vi "Soft_Robot Model Two States.vi"() -> ()   [LabVIEW 2015]
uses:
  <vilib>/addons/Control Design/_Model Construction/Model Typedefs.llb/CD State Space Model (MIMO).ctl
  <vilib>/addons/Control Design/_Model Construction/Model Typedefs.llb/CD General Elements.ctl
  <vilib>/Analysis/7linalg.llb/Create Special Real Matrix.vi
  <vilib>/addons/Control Design/_Model Construction/Model Creation.llb/Model Creation SubVI/cd_Create State Space Model.vi
  <vilib>/addons/Control Design/_State Feedback Control/State Feedback Control.llb/State Feedback Control SubVis/cd_Linear Quadratic Regulator.vi
  <vilib>/addons/Control Design/_Stochastic Systems/Stochastic Systems.llb/CD Construct Noise Model (Numeric).vi
  <vilib>/Simulation/Estimation/Implementation/NILVSim Discrete Kalman Filter.llb/SIM Disc KF Pred and Corr with Pred Gain with Checking Direct LV.vi
  <vilib>/FPGAPlugInAG/myRIO-1900/niLvFpga_Open_myRIO-1900.vi
  <vilib>/rvi/interface/common/dynamic/niFpgaDynamicAddResources.vi
  <vilib>/Utility/error.llb/Error Cluster From Error Code.vi
  <vilib>/rvi/errors/niLvFpgaAdjustHostInterfaceError.vi
  <vilib>/FPGAPlugInAG/Dynamic/niLvFpga_Close_Dynamic.vi
  <vilib>/Simulation/Implementation/XNodeFramework/SimXNode/SimX.xnode
  <vilib>/rvi/interface/nirviOpenFPGA/nirviOpenFPGA.xnode
  FPGA Bitfiles/ACC20115_FPGATarget_CurrentControlle_Dt5vFgOzYtY.lvbitx
  Current Controller.vi
  <vilib>/rvi/interface/nirviReadWriteControl/nirviReadWriteControl.xnode
  <vilib>/rvi/interface/nirviCloseFPGA/nirviCloseFPGA.xnode
  NiFpgaLv.dll
  <vilib>/rvi/interface/Simulation/niFpgaSimulationCallBeginRW.vi
  <vilib>/addons/Control Design/_Model Construction/NI_LinSys_Model Creation.lvlib
  <vilib>/addons/Control Design/_State Feedback Control/NI_CD_State Feedback Control.lvlib
  <vilib>/addons/Control Design/_Stochastic Systems/NI_CD_Stochastic Systems.lvlib
  <vilib>/Analysis/NI_AALPro.lvlib
  <vilib>/addons/Control Design/_Model Construction/NI_LinSys_Model Typedefs.lvlib
panel:
  in  "Stop":bool
  out "Fusion Data":dbl(graph)
  out "xhat(k+1|k) 2":dbl[](array[numeric])
  out "xhat(k|k) 2":dbl[](array[numeric])
  out "State-Space Model 2":T1 {"Transport Delay" format="%.2f"; "D" format="%#.2g"; "C" format="%#.2g"; "B" format="%#.2g"; "A" format="%#.2g"; "properties"."Sampling Time" format="%#.6p"; "properties"."Output Delays" format="%.4f"; "properties"."Input Delays" format="%.4f"}
  in  "C 2":dbl[][](array[numeric]) format="%#.5g"
  in  "B 2":dbl[][](array[numeric]) format="%#.5g"
  in  "A 2":dbl[][](array[numeric]) format="%#.5g"
  in  "LQR Output weighting matrix (R) 2":dbl[](array[slide])=[0.061359072734131735] scale=0.0001..10.0
  in  "LQR State Weight Matrix (Q) 2":dbl[](array[slide])=[1.133823501217849, 15.19911082952933] scale=0.001..1000.0
  in  "Initial  Cov P(0|-1) 2":dbl[][](array[numeric])=[[1.0, 0.0], [0.0, 1.0]]
  in  "Initial  xhat(0|-1) 2":dbl[](array[numeric])=[1.0, 0.0]
  in  "KF R 2":dbl[][](array[numeric])=[[0.1]]
  in  "KF Q 2":dbl[][](array[numeric])=[[0.01, 0.0], [0.0, 0.001]]
  in  "SP1: 2":dbl(slide)=40.87020302841148 min=0.0 max=0.0 scale=0.0..720.0
  out "KF estimate 2":dbl[](graph)
  in  "D 2":dbl[][](array[numeric]) format="%#.5g"
  out "xhat(k+1|k)":dbl[](array[numeric])
  in  "Tab Control":enum32{"Outputs/Control", "Model Info"}(tab)
  out "DAC Inlet Valve 2":i32(graph)
  out "Fusion Data":dbl(graph)
  out "KF estimate":dbl[](graph)
  in  "SP1:":dbl(slide)=40.87020302841148 min=0.0 max=0.0 scale=0.0..720.0
  in  "Stop":bool
  out "Status?":bool
  in  "Current (mA)":i32
  out "error out":errorcluster
  out "xhat(k|k)":dbl[](array[numeric])
  in  "D":dbl[][](array[numeric]) format="%#.5g"
  in  "KF Q":dbl[][](array[numeric])=[[0.01, 0.0], [0.0, 0.001]]
  in  "KF R":dbl[][](array[numeric])=[[0.1]]
  in  "Initial  xhat(0|-1)":dbl[](array[numeric])=[1.0, 0.0]
  in  "Initial  Cov P(0|-1)":dbl[][](array[numeric])=[[1.0, 0.0], [0.0, 1.0]]
  in  "LQR State Weight Matrix (Q)":dbl[](array[slide])=[1.133823501217849, 15.19911082952933] scale=0.001..1000.0
  in  "LQR Output weighting matrix (R)":dbl[](array[slide])=[0.061359072734131735] scale=0.0001..10.0
  in  "A":dbl[][](array[numeric]) format="%#.5g"
  in  "B":dbl[][](array[numeric]) format="%#.5g"
  in  "C":dbl[][](array[numeric]) format="%#.5g"
  out "State-Space Model":T1 {"Transport Delay" format="%.2f"; "D" format="%#.2g"; "C" format="%#.2g"; "B" format="%#.2g"; "A" format="%#.2g"; "properties"."Sampling Time" format="%#.6p"; "properties"."Output Delays" format="%.4f"; "properties"."Input Delays" format="%.4f"}
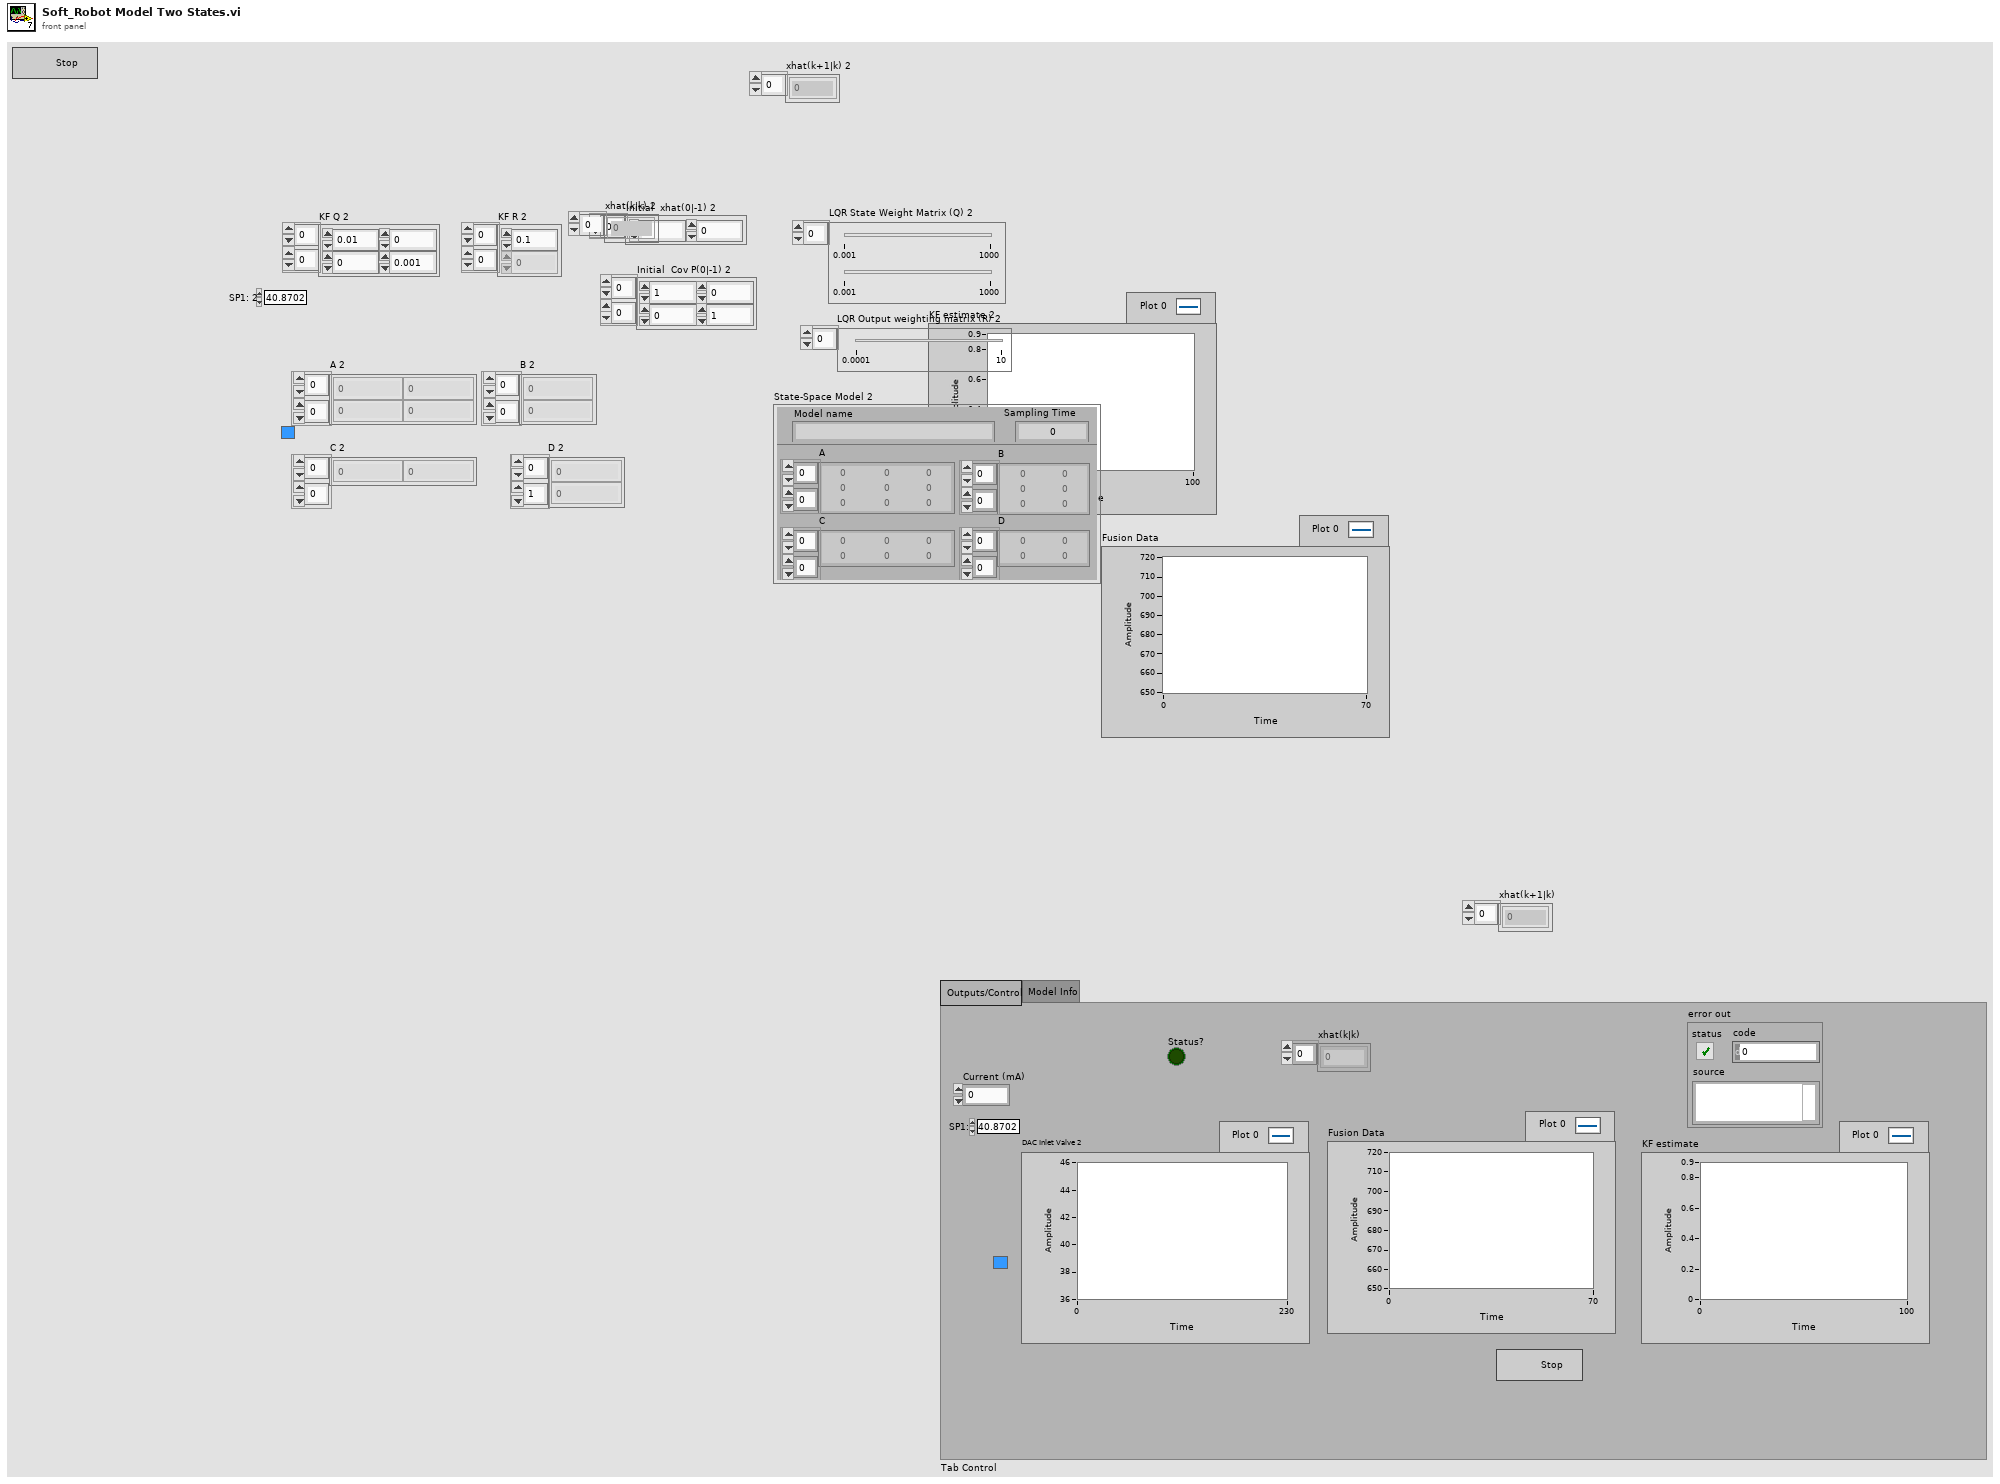
[diagram p1: front panel]
types:
  T1 = typedef "NI_LinSys_Model Typedefs.lvlib/CD State Space Model (MIMO).ctl" = cluster{"properties":T2, "A":dbl[][], "B":dbl[][], "C":dbl[][], "D":dbl[][], "StateNames":string[], "Transport Delay":dbl[][]}
  T2 = typedef "NI_LinSys_Model Typedefs.lvlib/CD General Elements.ctl" = cluster{"Model name":string, "Input names":string[], "Output names":string[], "Input Delays":dbl[], "Output Delays":dbl[], "Sampling Time":dbl, "Notes":string}
  T3 = enum16{"state weighting", "output weighting, Dim Q = Ny", "output weighting, Dim Q = Nx"}
  T4 = enum32{"Identity", "Diagonal", "Toepliz", "Vandermonde", "Companion"}
  T5 = typedef "NI_Matrix.lvlib/RealMatrix.ctl" = dbl[][]
  T6 = typedef "NI_CD_Stochastic Systems.lvlib/cd_Stochastic State-Space Model.ctl" = cluster{"Sampling Time (s)":dbl, "G":dbl[][], "B":dbl[][], "A":dbl[][], "C":dbl[][], "D":dbl[][], "H":dbl[][]}
  T7 = typedef "NI_CD_Stochastic Systems.lvlib/cd_Second-Order Statistics Noise Model.ctl" = cluster{"Q":dbl[][], "E{w}":dbl[], "E{v}":dbl[], "R":dbl[][], "N":dbl[][]}
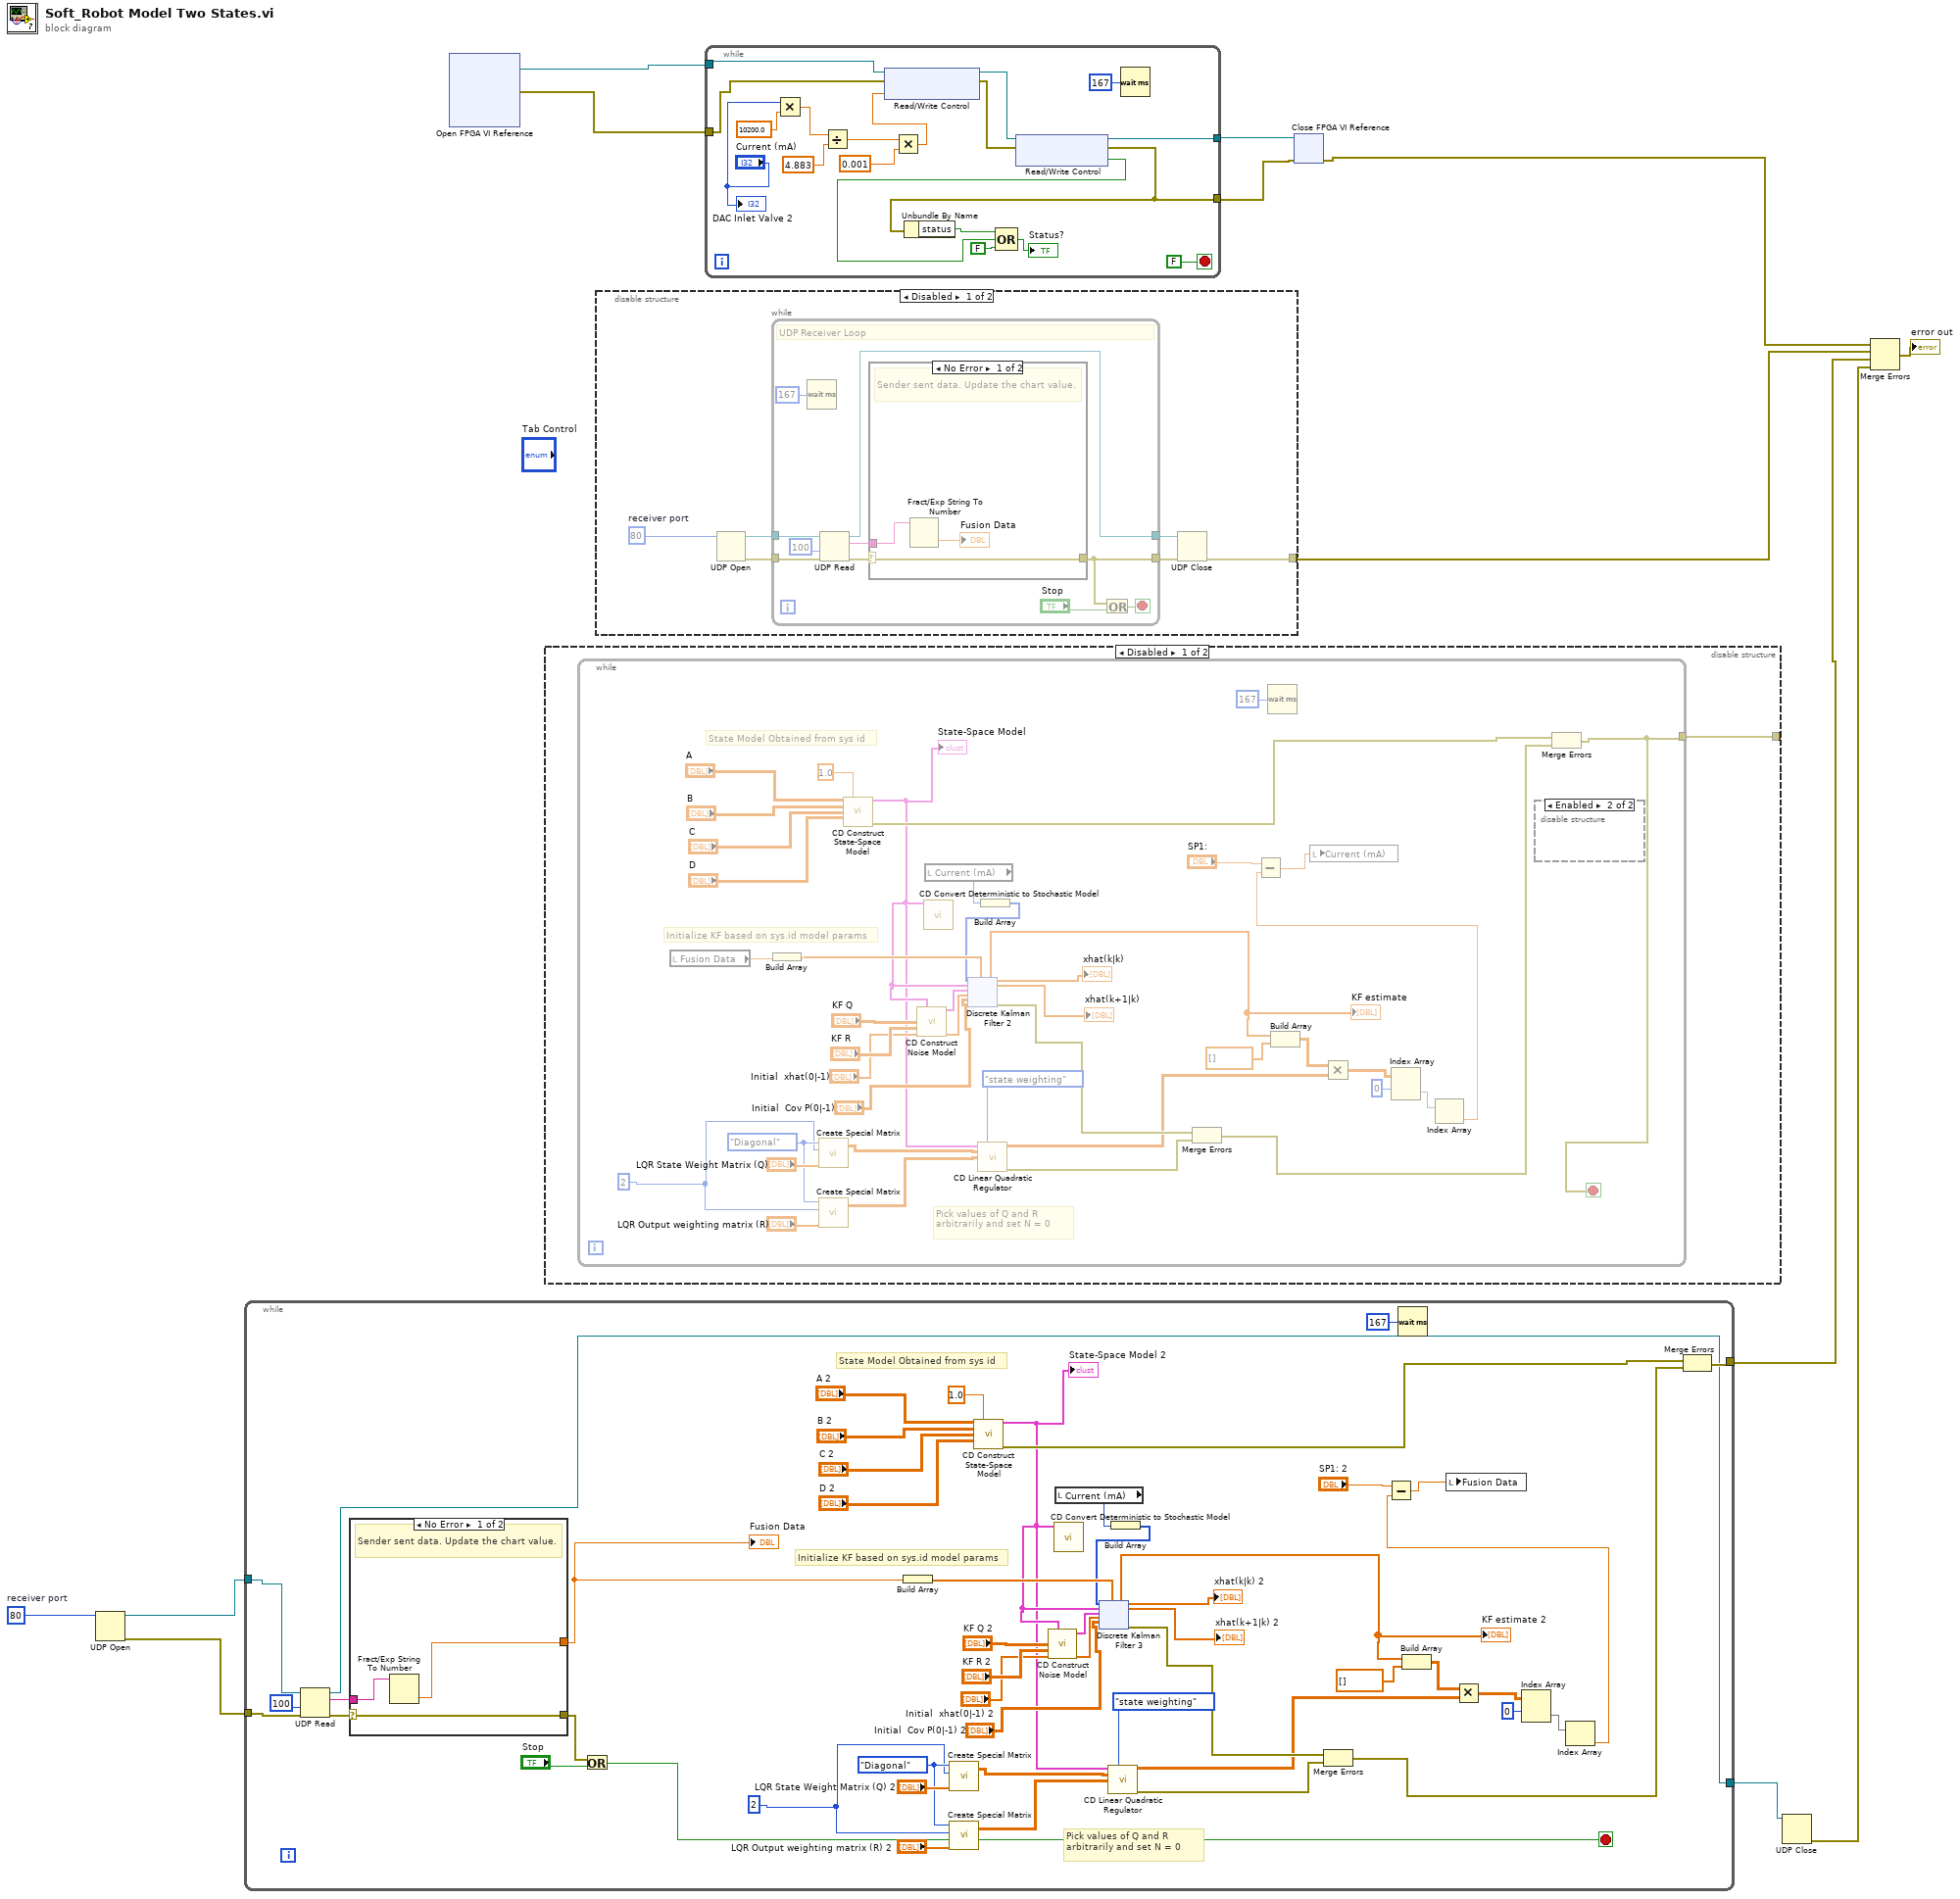
[diagram p0: block diagram]
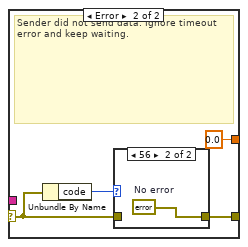
[diagram p2: hidden frame]
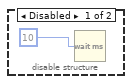
[diagram p4: hidden frame]
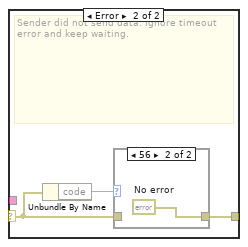
[diagram p6: hidden frame]
diagram:
  w6 = u16 80  # receiver port
  n1 = UDP Open(11:w6) -> (port=w5:refnum<k16>, 0:w4:errorcluster)  [unwired: 4 in, 1 out]
  n2 = while {
    tunnel: [w25] -> w1
    tunnel: w5 -> [w18]
    tunnel: w4 -> [w17]
    tunnel: [w14] -> w3
    stop <- w15 stop-if-true
    w35 = 2
    w42 = T4."Diagonal" ("matrix type")
    # "Pick values of Q and R\narbitrarily and set N = 0"
    # "State Model Obtained from sys id"
    # "Initialize KF based on sys.id model params"
    n3 = UDP Read(connection ID=w18, timeout ms (25000)=100, 8:w17) -> (data out=w21:string, error out=w20:errorcluster, 3:w14:refnum<k16>)  [unwired: 3 out]
    n4 = case shown="No Error" w20 {
      selector: w20 -> [w65 w69]
      tunnel: w21 -> [w66 _]
      tunnel: [w65 w68] -> w19
      tunnel: [w64 0.0] -> w16
      frame No Error {
        # "Sender sent data. Update the chart value."
        n5 = Fract/Exp String To Number(string=w66) -> (number=w64:dbl)  [unwired: 3 in, 1 out]
      }
      frame Error {
        # "Sender did not send data. Ignore timeout error and keep waiting."
        n6 = Unbundle By Name(w69) -> ("code"=w70:i32)
        n7 = case shown="56" w70 {
          tunnel: w69 -> [w71 _]
          tunnel: [w71 w72] -> w68
          frame Default {
          }
          frame 56 {
            w72 = errorcluster {"status"=FALSE, "code"=0, "source"=""}  # No error
          }
        }
      }
    }
    "Fusion Data" <- w16
    n8 = Or(x=w19, y="Stop") -> (x .or. y?=w15:bool)
    n9 = Build Array ("Build Array 6")(w16) -> (w53:dbl[])
    n10 = call-poly <vilib>:"Create Special Matrix.vi"("matrix type"=w42, "matrix size"=w35, "Input Vector1"="LQR State Weight Matrix (Q) 2") -> ("Special Matrix"=w39:T5)  [unwired: 2 in, 1 out]
    n11 = call-poly <vilib>:"Create Special Matrix.vi"("matrix type"=w42, "matrix size"=w35, "Input Vector1"="LQR Output weighting matrix (R) 2") -> ("Special Matrix"=w38:T5)  [unwired: 2 in, 1 out]
    n12 = call-poly <vilib>:"CD Construct State-Space Model.vi"("A"="A 2", "Sampling Time (s)"=1.0, "B"="B 2", "C"="C 2", "D"="D 2") -> ("State-Space Model"=w40:T1, "error out"=w54:errorcluster)  [unwired: 9 in]
    "State-Space Model 2" <- w40
    n13 = call <vilib>:"CD Convert Deterministic to Stochastic Model.vi"("Deterministic State-Space Model"=w40) -> ("Stochastic State-Space Model"=w49:T6)  [unwired: 13 in, 1 out]
    n14 = call-poly <vilib>:"CD Construct Noise Model.vi"("Stochastic State-Space Model"=w49, "Q"="KF Q 2", "R"="KF R 2") -> ("Second-Order Statistics Noise Model out"=w29:T7)  [unwired: 11 in, 1 out]
    n15 = local read "Current (mA)"() -> (w55:i32)
    n16 = call-poly <vilib>:"CD Linear Quadratic Regulator.vi"("State-Space Model"=w40, "Weighting Type"=T3."state weighting", "Q"=w39, "R"=w38) -> ("Optimal Gain (K)"=w37:dbl[][], "error out"=w36:errorcluster)  [unwired: 8 in, 2 out]
    n17 = Build Array ("Build Array 5")(w55) -> (w45:i32[])
    n18 = xnode ("Discrete Kalman Filter 3")("input u(k)"=w45, "Stochastic State-Space Model"=w49, "Second-Order Statistics Noise Model"=w29, "Initial State Estimate xhat(0|-1)"="Initial  xhat(0|-1) 2", "Initial Estimation Error Covariance P(0|-1)"="Initial  Cov P(0|-1) 2", "Output y(k)"=w53) -> ("Estimated Output yhat(k)"=w52:dbl[], "Corrected State Estimate xhat(k|k)"=→"xhat(k|k) 2":dbl[], "Predicted State Estimate xhat(k+1|k)"=→"xhat(k+1|k) 2":dbl[], "error out"=w51:errorcluster)  [unwired: 2 in, 4 out]
    "KF estimate 2" <- w52
    n19 = Merge Errors(w51, w36) -> (w24:errorcluster)
    n20 = Wait (ms)(milliseconds to wait=u32 167) -> ()  [unwired: 1 out]
    n21 = Build Array ("Build Array 9")(w52, dbl[] [] ("element")) -> (w59:dbl[][])
    n22 = Multiply(x=w59, y=w37) -> (x*y=w61:dbl[][])
    n23 = Index Array(array=w61, index (row)=0) -> (element=w63:dbl[])  [unwired: 1 in]
    n24 = Index Array ("Index Array 2")(array=w63) -> (element=w56:dbl)  [unwired: 1 in]
    n25 = Subtract(x="SP1: 2", y=w56) -> (x-y=w26:dbl)
    n26 = local write "Fusion Data"(w26) -> ()
    n27 = Merge Errors(w54, w24) -> (w25:errorcluster)
  }
  n28 = xnode "Open FPGA VI Reference"() -> ("FPGA VI Reference Out"=w7:refnum<k20>, "error out"=w8:errorcluster)  [unwired: 2 in]
  n29 = disable-structure shown="Disabled" {
    disable-tunnel: [w89 _] -> _
    frame Disabled {
      n30 = while {
        tunnel: [w98] -> w89
        stop <- w98 stop-if-true
        w99 = 2
        w106 = T4."Diagonal" ("matrix type")
        # "Pick values of Q and R\narbitrarily and set N = 0"
        # "State Model Obtained from sys id"
        # "Initialize KF based on sys.id model params"
        n31 = local read "Fusion Data"() -> (w121:dbl)
        n32 = Build Array ("Build Array 6")(w121) -> (w117:dbl[])
        n33 = call-poly <vilib>:"Create Special Matrix.vi"("matrix type"=w106, "matrix size"=w99, "Input Vector1"="LQR State Weight Matrix (Q)") -> ("Special Matrix"=w103:T5)  [unwired: 2 in, 1 out]
        n34 = call-poly <vilib>:"Create Special Matrix.vi"("matrix type"=w106, "matrix size"=w99, "Input Vector1"="LQR Output weighting matrix (R)") -> ("Special Matrix"=w102:T5)  [unwired: 2 in, 1 out]
        n35 = call-poly <vilib>:"CD Construct State-Space Model.vi"("A"="A", "Sampling Time (s)"=1.0, "B"="B", "C"="C", "D"="D") -> ("State-Space Model"=w104:T1, "error out"=w118:errorcluster)  [unwired: 9 in]
        "State-Space Model" <- w104
        n36 = call <vilib>:"CD Convert Deterministic to Stochastic Model.vi"("Deterministic State-Space Model"=w104) -> ("Stochastic State-Space Model"=w113:T6)  [unwired: 13 in, 1 out]
        n37 = call-poly <vilib>:"CD Construct Noise Model.vi"("Stochastic State-Space Model"=w113, "Q"="KF Q", "R"="KF R") -> ("Second-Order Statistics Noise Model out"=w92:T7)  [unwired: 11 in, 1 out]
        n38 = local read "Current (mA)"() -> (w119:i32)
        n39 = call-poly <vilib>:"CD Linear Quadratic Regulator.vi"("State-Space Model"=w104, "Weighting Type"=T3."state weighting", "Q"=w103, "R"=w102) -> ("Optimal Gain (K)"=w101:dbl[][], "error out"=w100:errorcluster)  [unwired: 8 in, 2 out]
        n40 = Build Array ("Build Array 5")(w119) -> (w109:i32[])
        n41 = xnode ("Discrete Kalman Filter 2")("input u(k)"=w109, "Stochastic State-Space Model"=w113, "Second-Order Statistics Noise Model"=w92, "Initial State Estimate xhat(0|-1)"="Initial  xhat(0|-1)", "Initial Estimation Error Covariance P(0|-1)"="Initial  Cov P(0|-1)", "Output y(k)"=w117) -> ("Estimated Output yhat(k)"=w116:dbl[], "Corrected State Estimate xhat(k|k)"=→"xhat(k|k)":dbl[], "Predicted State Estimate xhat(k+1|k)"=→"xhat(k+1|k)":dbl[], "error out"=w115:errorcluster)  [unwired: 2 in, 4 out]
        "KF estimate" <- w116
        n42 = Merge Errors(w115, w100) -> (w124:errorcluster)
        n43 = Wait (ms)(milliseconds to wait=u32 167) -> ()  [unwired: 1 out]
        n44 = Build Array ("Build Array 9")(w116, dbl[] [] ("element")) -> (w126:dbl[][])
        n45 = Multiply(x=w126, y=w101) -> (x*y=w128:dbl[][])
        n46 = Index Array(array=w128, index (row)=0) -> (element=w130:dbl[])  [unwired: 1 in]
        n47 = Index Array ("Index Array 2")(array=w130) -> (element=w122:dbl)  [unwired: 1 in]
        n48 = Subtract(x="SP1:", y=w122) -> (x-y=w120:dbl)
        n49 = local write "Current (mA)"(w120) -> ()
        n50 = disable-structure shown="Enabled" {
          frame Disabled {
            n51 = Wait (ms)(milliseconds to wait=u32 10 ("millisecond timer value")) -> ()  [unwired: 1 out]
          }
          frame Enabled {
          }
        }
        n52 = Merge Errors(w118, w124) -> (w98:errorcluster)
      }
    }
    frame Enabled {
    }
  }
  n53 = disable-structure shown="Disabled" {
    disable-tunnel: [w148 _] -> w10
    frame Disabled {
      w149 = u16 80  # receiver port
      n54 = UDP Open(11:w149) -> (port=w150:refnum<k16>, 0:w151:errorcluster)  [unwired: 4 in, 1 out]
      n55 = while {
        tunnel: w150 -> [w163]
        tunnel: [w155] -> w153
        tunnel: w151 -> [w160]
        tunnel: [w156] -> w152
        stop <- w161 stop-if-true
        # "UDP Receiver Loop"
        n56 = Wait (ms)(milliseconds to wait=u32 167) -> ()  [unwired: 1 out]
        n57 = UDP Read(connection ID=w163, timeout ms (25000)=100, 8:w160) -> (data out=w158:string, error out=w157:errorcluster, 3:w155:refnum<k16>)  [unwired: 3 out]
        n58 = case shown="No Error" w157 {
          selector: w157 -> [w164 w168]
          tunnel: w158 -> [w166 _]
          tunnel: [w164 w167] -> w156
          frame No Error {
            # "Sender sent data. Update the chart value."
            n59 = Fract/Exp String To Number(string=w166) -> (number=→"Fusion Data":dbl)  [unwired: 3 in, 1 out]
          }
          frame Error {
            # "Sender did not send data. Ignore timeout error and keep waiting."
            n60 = Unbundle By Name(w168) -> ("code"=w169:i32)
            n61 = case shown="56" w169 {
              tunnel: w168 -> [w170 _]
              tunnel: [w170 w171] -> w167
              frame Default {
              }
              frame 56 {
                w171 = errorcluster {"status"=FALSE, "code"=0, "source"=""}  # No error
              }
            }
          }
        }
        n62 = Or(x=w156, y="Stop") -> (x .or. y?=w161:bool)
      }
      n63 = UDP Close(connection ID=w153, 8:w152) -> (error out=w148:errorcluster)  [unwired: 1 out]
    }
    frame Enabled {
    }
  }
  n64 = while {
    tunnel: w7 -> [w189]
    tunnel: w8 -> [w173]
    tunnel: [w183] -> w12
    tunnel: [w181] -> w13
    stop <- FALSE stop-if-true
    n65 = Multiply(x="Current (mA)", y=10200.0) -> (x*y=w176:dbl)
    n66 = Divide(x=w176, y=4.883) -> (x/y=w179:dbl)
    n67 = Multiply(x=w179, y=0.001) -> (x*y=w175:dbl)
    n68 = xnode "Read/Write Control"("FPGA VI Reference In"=w189, "error in"=w173, "DAC Inlet Valve"=w175) -> ("FPGA VI Reference Out"=w188:refnum<k20>, "error out"=w187:errorcluster)
    n69 = xnode "Read/Write Control"("FPGA VI Reference In"=w188, "error in"=w187) -> ("FPGA VI Reference Out"=w181:refnum<k20>, "error out"=w183:errorcluster, "Inlet Overflow?"=w182:bool)
    n70 = Unbundle By Name(w183) -> ("status"=w185:bool)
    n71 = Compound Arithmetic op=OR(w185, w182, FALSE ("value")) -> (→"Status?":bool)
    n72 = Wait (ms)(milliseconds to wait=u32 167) -> ()  [unwired: 1 out]
    "DAC Inlet Valve 2" <- "Current (mA)"
  }
  n73 = xnode "Close FPGA VI Reference"("FPGA VI Reference In"=w13, "error in"=w12) -> ("error out"=w11:errorcluster)
  n74 = UDP Close(connection ID=w3) -> (error out=w2:errorcluster)  [unwired: 1 in, 1 out]
  n75 = Merge Errors(w11, w10, w1, w2) -> (→"error out":errorcluster)
